vi "Init.vi"(10 "Player ID":i32, 11 "TeamEffort in":refnum<class "TeamEffort.lvclass">) -> (3 "TeamEffort out":refnum<class "TeamEffort.lvclass">)   [LabVIEW 2015, in "TeamEffort.lvclass"]
uses:
  TeamEffort.lvclass
  Grid Cluster.ctl
  Player Cluster.ctl
  Type Defs/Action Enum.ctl
  Type Defs/Direction Enum.ctl
  Square/Square.lvclass
  Square/Square.lvclass/Square.ctl
  TeamEffort.lvclass/TeamEffort.ctl
  Square/Read Board Size.vi
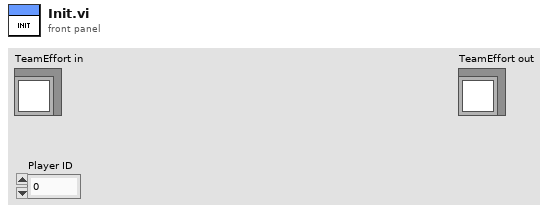
[diagram p1: front panel]
types:
  T1 = typedef "TeamEffort.lvclass/Player Cluster.ctl" = cluster{"Player #":i32, "Exp. Move":i32, "X":i16, "Y":i16, "Action":T2, "Direction":T3, "Moved?":bool, "Replicated":refnum<class "Square.lvclass">}
  T2 = typedef "Square.lvclass/Action Enum.ctl" = enum16{"Wait", "Move", "Attack", "Replicate"}
  T3 = typedef "Square.lvclass/Direction Enum.ctl" = enum16{"NW", "N", "NE", "E", "SE", "S", "SW", "W"}
  T4 = typedef "TeamEffort.lvclass/Grid Cluster.ctl" = cluster{"p[x][y]":i32[][], "Move Count":i32, "Info[p]":T1[]}
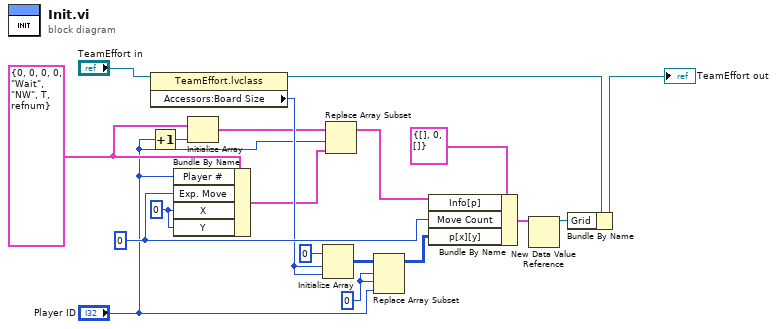
[diagram p0: block diagram]
diagram:
  w9 = 0
  w5 = T1 {"Player #"=0, "Exp. Move"=0, "X"=0, "Y"=0, "Action"=enum."Wait", "Direction"=enum."NW", "Moved?"=TRUE, "Replicated"=refnum} ("Player Info")
  w17 = i16 0 ("index (row)")
  w18 = 0 ("Move Count")
  n1 = Increment(x="Player ID") -> (x+1=w6:i32)
  n2 = property class="TeamEffort.lvclass"(reference="TeamEffort in") -> (reference out=w14:refnum<class "TeamEffort.lvclass">, "Accessors:Board Size"=w12:i32)  [unwired: 1 in, 1 out]
  n3 = Bundle By Name(cluster=w5, "Player #"="Player ID", "Exp. Move"=w18, "X"=w17, "Y"=w17) -> (w3:T1)
  n4 = Initialize Array(w5, w6) -> (w4:T1[])
  n5 = Initialize Array(0, w12, w12) -> (w11:i32[][])
  n6 = Replace Array Subset(array=w4, new element=w3, index="Player ID") -> (w2:T1[])
  n7 = Replace Array Subset(array=w11, new element="Player ID", index (row)=w9, index (col)=w9) -> (w10:i32[][])
  n8 = Bundle By Name(cluster=T4 {"p[x][y]"=[], "Move Count"=0, "Info[p]"=[]} ("Grid"), "Info[p]"=w2, "Move Count"=w18, "p[x][y]"=w10) -> (w16:T4)
  n9 = New Data Value Reference(data value=w16) -> (data value reference=w15:refnum<data-value>)  [unwired: 1 in, 1 out]
  n10 = Bundle By Name(cluster=w14, "Grid"=w15) -> (→"TeamEffort out":refnum<class "TeamEffort.lvclass">)
